vi "Configure IQ Correction.vi"(8 "error in (no error)":errorcluster, 10 "Optimized Path (0: RF Output)":u16(ring) items=["RF Output", "External"], 11 "VISA resource name":refnum<visa-resource-name>) -> (0 "error out":errorcluster, 3 "VISA resource name out":refnum<visa-resource-name>)   [LabVIEW 2009, in "Agilent PSG MXG Series.lvlib"]
doc: "Configures the I/Q correction optimized path.\n\n<B>Notes:</B>\n(1) This VI is valid only in N5182A."
uses:
  Agilent PSG MXG Series.lvlib
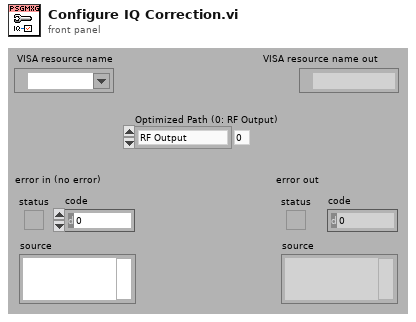
[diagram p1: front panel]
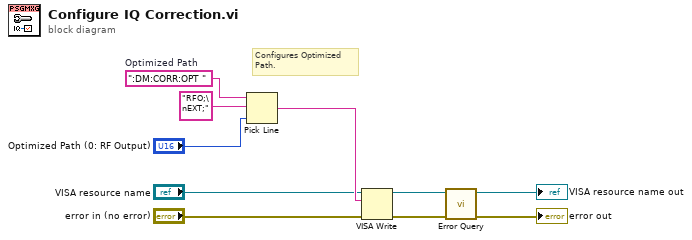
[diagram p0: block diagram]
diagram:
  w10 = ":DM:CORR:OPT "  # Optimized Path
  # "Configures Optimized\nPath."
  n1 = Pick Line(string ("")=w10, multi-line string="RFO;\nEXT;", line index="Optimized Path (0: RF Output)") -> (output string=w7:string)
  n2 = VISA Write(VISA resource name="VISA resource name", write buffer=w7, error in (no error)="error in (no error)") -> (VISA resource name out=w6:refnum<visa-resource-name>, error out=w5:errorcluster)  [unwired: 1 out]
  n3 = call "Error Query.vi"("error in (no error)"=w5, "VISA resource name"=w6) -> ("error out"=→"error out":errorcluster, "VISA resource name out"=→"VISA resource name out":refnum<visa-resource-name>)  [unwired: 8 out]
